vi "Устройство ввода.vi"(1 "Reset":bool, 2 "c":bool, 3 "Keyboard":T2, 4 "Minus":bool) -> (0 "N":T1)   [LabVIEW 2013]
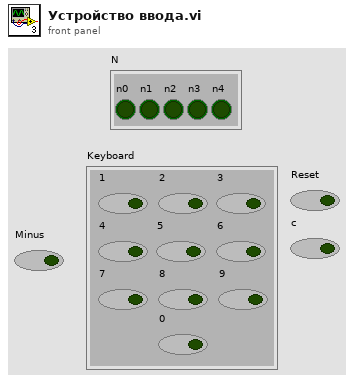
[diagram p1: front panel]
types:
  T1 = cluster{"n0":bool, "n1":bool, "n2":bool, "n3":bool, "n4":bool}
  T2 = cluster{"0":bool, "1":bool, "2":bool, "3":bool, "4":bool, "5":bool, "6":bool, "7":bool, "8":bool, "9":bool}
  T3 = cluster{"x0":bool, "x1":bool, "x2":bool, "x3":bool}
  T4 = cluster{"q3":bool, "q2":bool, "q1":bool, "q0":bool}
  T5 = cluster{"q0":bool, "q1":bool, "q2":bool, "q3":bool}
  T6 = cluster{"r4":bool, "r3":bool, "r2":bool, "r1":bool, "r0":bool}
  T7 = cluster{"r0":bool, "r1":bool, "r2":bool, "r3":bool, "r4":bool}
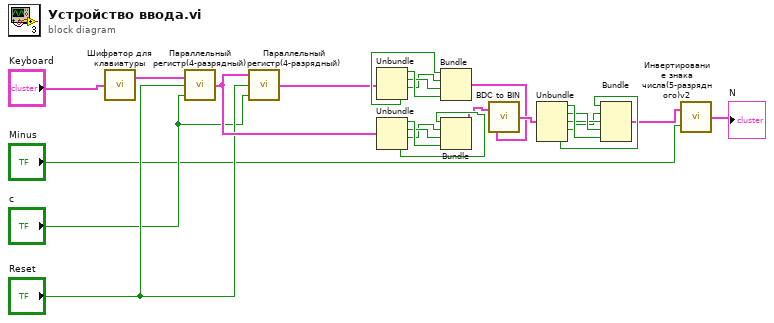
[diagram p0: block diagram]
diagram:
  n1 = call "Шифратор для клавиатуры.vi"("Keyboard"="Keyboard") -> ("Bin"=w13:T3)  [unwired: 1 out]
  n2 = call "Параллельный регистр(4-разрядный).vi"("C"="c", "Reset"="Reset", "Cluster"=w13) -> ("output cluster"=w16:T4)
  n3 = call "Параллельный регистр(4-разрядный).vi"("C"="c", "Reset"="Reset", "Cluster"=w16) -> ("output cluster"=w15:T4)
  n4 = Unbundle(w15) -> ("q3"=w20:bool, "q2"=w19:bool, "q1"=w18:bool, "q0"=w17:bool)
  n5 = Unbundle(w16) -> ("q3"=w24:bool, "q2"=w23:bool, "q1"=w22:bool, "q0"=w21:bool)
  n6 = Bundle("q0"=w17, "q1"=w18, "q2"=w19, "q3"=w20) -> (w5:T5)  [unwired: 1 in]
  n7 = Bundle("q0"=w21, "q1"=w22, "q2"=w23, "q3"=w24) -> (w6:T5)  [unwired: 1 in]
  n8 = call "BDC to BIN.vi"("BDC0"=w5, "BDC1"=w6) -> ("R"=w12:T6)
  n9 = Unbundle(w12) -> ("r4"=w11:bool, "r3"=w10:bool, "r2"=w9:bool, "r1"=w8:bool, "r0"=w7:bool)
  n10 = Bundle("r0"=w7, "r1"=w8, "r2"=w9, "r3"=w10, "r4"=w11) -> (w2:T7)  [unwired: 1 in]
  n11 = call "Инвертирование знака числа(5-разрядного)v2.vi"("sign"="Minus", "A"=w2) -> ("R"=→"N":T7)
